vi "Add Status Section.vi"(8 "error in":errorcluster, 11 "custom device in":T1 format="%.0x") -> (0 "error out":errorcluster, 2 "status section":T1 format="%.0x", 3 "custom device out":T1 format="%.0x")   [LabVIEW 2020, in "AIM MIL-STD-1553 Scripting.lvlib"]
uses:
  AIM MIL-STD-1553 Scripting.lvlib
  <vilib>/NI VeriStand/Custom Device API/Custom Device API.lvlib
  Constants.vi
  <vilib>/NI VeriStand/Custom Device API/Custom Device Item Ref.ctl
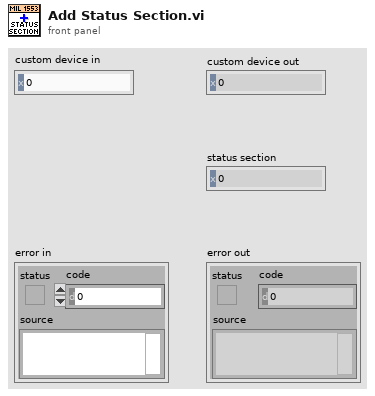
[diagram p1: front panel]
types:
  T1 = typedef "Custom Device API.lvlib/Custom Device Item Ref.ctl" = u64
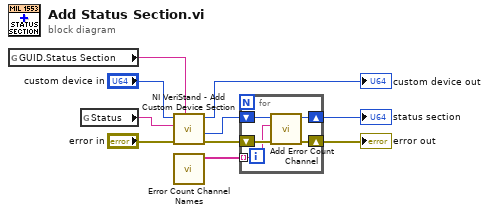
[diagram p0: block diagram]
diagram:
  n1 = global read "Constants.vi" "GUID.Status Section"() -> (w7:string)
  n2 = global read "Constants.vi" "Status"() -> (w6:string)
  n3 = call <vilib>:"NI VeriStand - Add Custom Device Section.vi"("GUID (Default Section)"=w7, "error in (no error)"="error in", "Section Name"=w6, "Parent Ref in"="custom device in") -> ("error out"=w5:errorcluster, "Section Ptr"=w2:T1, "Parent Ref out"=→"custom device out":T1)  [unwired: 4 in, 1 out]
  n4 = call "Error Count Channel Names.vi"() -> ("error count channel names"=w3:string[])  [unwired: 11 in]
  n5 = for {
    shift-right: [w13] -> w4
    shift-left: w5 -> [w14]
    tunnel: w3 -> [w12] mode=indexing
    shift-right: [w11] -> w1
    shift-left: w2 -> [w15]
    n6 = call "Add Error Count Channel.vi"("error in"=w14, "error count channel name"=w12, "status section in"=w15) -> ("error out"=w13:errorcluster, "status section out"=w11:T1)  [unwired: 6 in, 1 out]
  }
  "error out" <- w4
  "status section" <- w1
